vi "CH_LM Calibration Example.vi"() -> ()   [LabVIEW 2012, in "CH_LM.lvlib"]
doc: "This example VI can be used to query or set the calibration paramters."
uses:
  CH_LM.lvlib
  <vilib>/Utility/error.llb/DialogType.ctl
  CH_LM Calibration SlowADC Channel.ctl
  CH_LM ProbeQualifier.ctl
  CH_LM ProbeType.ctl
  CH_LM Meter Type.ctl
  CH_LM System StatusCluster.ctl
  CH_LM Date Format.ctl
panel:
  in  "Update All":bool
  in  "stop":bool
  in  "Unlock? (True)":bool
  out "GUI Loop":i32
  out "Lock timed out":bool
  in  "Reset Error":bool
  out "Event error":errorcluster
  in  "Tab Control":enum32{"Main", "Calibration"}(tab)
  out "Qualifier":T1
  out "Serial Number":string
  out "Head Temperature":dbl[unit]=273.15
  out "Status Description":string
  out "Status":T2
  out "Date Format":T3
  out "Time Stamp":timestamp format="%<%X\n%x>T"
  in  "Update Probe":bool
  out "Responsitivity":dbl format="%#.1g"
  out "Calibration Date":timestamp format="%<%x>T"
  out "Serial Number":string
  out "Probe Type":T4
  out "Probe Model":string
  out "Meter Type":T5
  out "Calibration Date":string
  out "Self-Test Result Message":string
  out "Self-Test Result Code":i32
  out "Date":string
  out "Revision":string
  out "Instrument Driver Revision":string
  out "Vendor":string
  out "Module":string
  out "timed out?":bool
  in  "Address":i32=1
  in  "Serial Number":string
  in  "Reset? (F: No)":bool
  in  "ID Query? (T: Yes)":bool
  in  "PYRO DAC Offset (0)":u16
  out "PYRO DAC Offset":u16
  in  "set Gain & Offset":bool
  in  "read Gain & Offset":bool
  in  "Hardware Calibration":T6={"Pyro DAC Attenuator"=0, "Pyro Input Attenuator"=1, "T Control"=0, "S Control"=0, "G Control"=0, "P Control"=0}
  in  "RTTR":u32=4294967295 format="%.0x"
  in  "Counts at 4V":i32
  in  "Counts at 0V":i32
  in  "DAC counts":i32
  out "Slow ADC value":i32 format="%.0x"
  in  "Slow ADC Channel":T7
  out "ADC value":i32 format="%.0x"
  out "Peak value":i32 format="%.0x"
  in  "set Probe Type":bool
  in  "Responsitivity new":dbl format="%#.1g"
  in  "Probe Type new":T4
  in  "Meter Info":bool
  in  "Calibration Date new":string
  in  "Serial Number new":string
  in  "Meter Type new":T5
  in  "Password":string
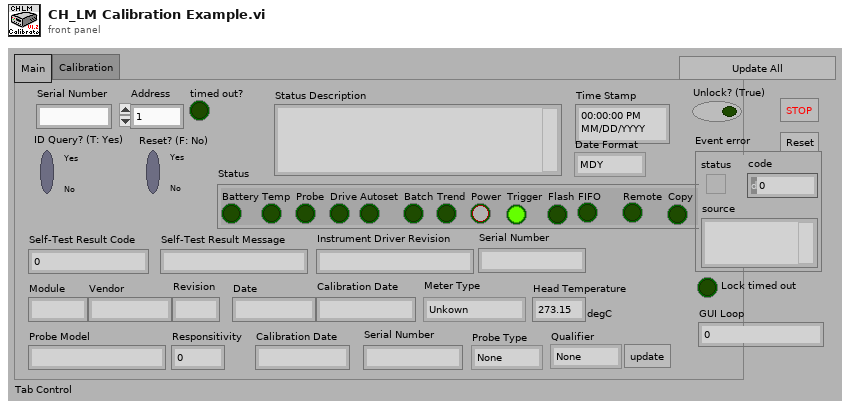
[diagram p1: front panel]
types:
  T1 = typedef "CH_LM.lvlib/CH_LM ProbeQualifier.ctl" = enum16{"None", "Single", "Quad", "No Spec"}
  T2 = typedef "CH_LM.lvlib/CH_LM System StatusCluster.ctl" = cluster{"Battery":bool, "Temp":bool, "Probe":bool, "Drive":bool, "Autoset":bool, "Batch":bool, "Trend":bool, "Power":bool, "Trigger":bool, "Flash":bool, "FIFO":bool, "Remote":bool, "Copy":bool}
  T3 = typedef "CH_LM.lvlib/CH_LM Date Format.ctl" = enum16{"MDY", "DMY"}
  T4 = typedef "CH_LM.lvlib/CH_LM ProbeType.ctl" = enum16{"None", "Thermopile", "Pyroelectric", "Optical"}
  T5 = typedef "CH_LM.lvlib/CH_LM Meter Type.ctl" = enum16{"Unkown", "TOP", "TO"}
  T6 = cluster{"Pyro DAC Attenuator":i32, "Pyro Input Attenuator":i32, "T Control":i32, "S Control":i32, "G Control":i32, "P Control":i32}
  T7 = typedef "CH_LM.lvlib/CH_LM Calibration SlowADC Channel.ctl" = enum16{"Up", "Down", "Left", "Right", "P Max", "L Thermistor", "P Thermistor", "Optical"}
  T8 = typedef "CH_LM.lvlib/CH_LM Calibration Hardware Override.ctl" = cluster{"Pyro DAC Attenuator":i32, "Pyro Input Attenuator":i32, "Q Control":i32, "S Control":i32, "G Control":i32, "P Control":i32}
  T9 = typedef "DialogType.ctl" = u16
  T10 = typedef "CH_LM.lvlib/CH_LM Calibration Data Thermopile.ctl" = cluster{"Range 1.0":T11}
  T11 = typedef "CH_LM.lvlib/CH_LM Calibration Data.ctl" = cluster{"Gain":dbl, "Offset":dbl}
  T12 = typedef "CH_LM.lvlib/CH_LM Calibration Data Pyroelectric.ctl" = cluster{"Range 0.1":T11, "Range 0.2":T11, "Range 0.4":T11, "Range 0.5":T11, "Range 0.8":T11, "Range 1.0":T11, "Range 2.0":T11, "Range 4.0":T11, "Range 5.0":T11, "Range 8.0":T11, "Range 10.0":T11, "Range 20.0":T11, "Range 40.0":T11, "Range 50.0":T11, "Range 80.0":T11, "Range 100.0":T11, "Range 200.0":T11, "Range 400.0":T11, "Range 500.0":T11, "Range 800.0":T11, "Range 1000.0":T11, "Range 2000.0":T11, "Range 4000.0":T11}
  T13 = typedef "CH_LM.lvlib/CH_LM Calibration Data Optical.ctl" = cluster{"Range 68.1 Ohm":T11, "Range 100.0 kOhm":T11}
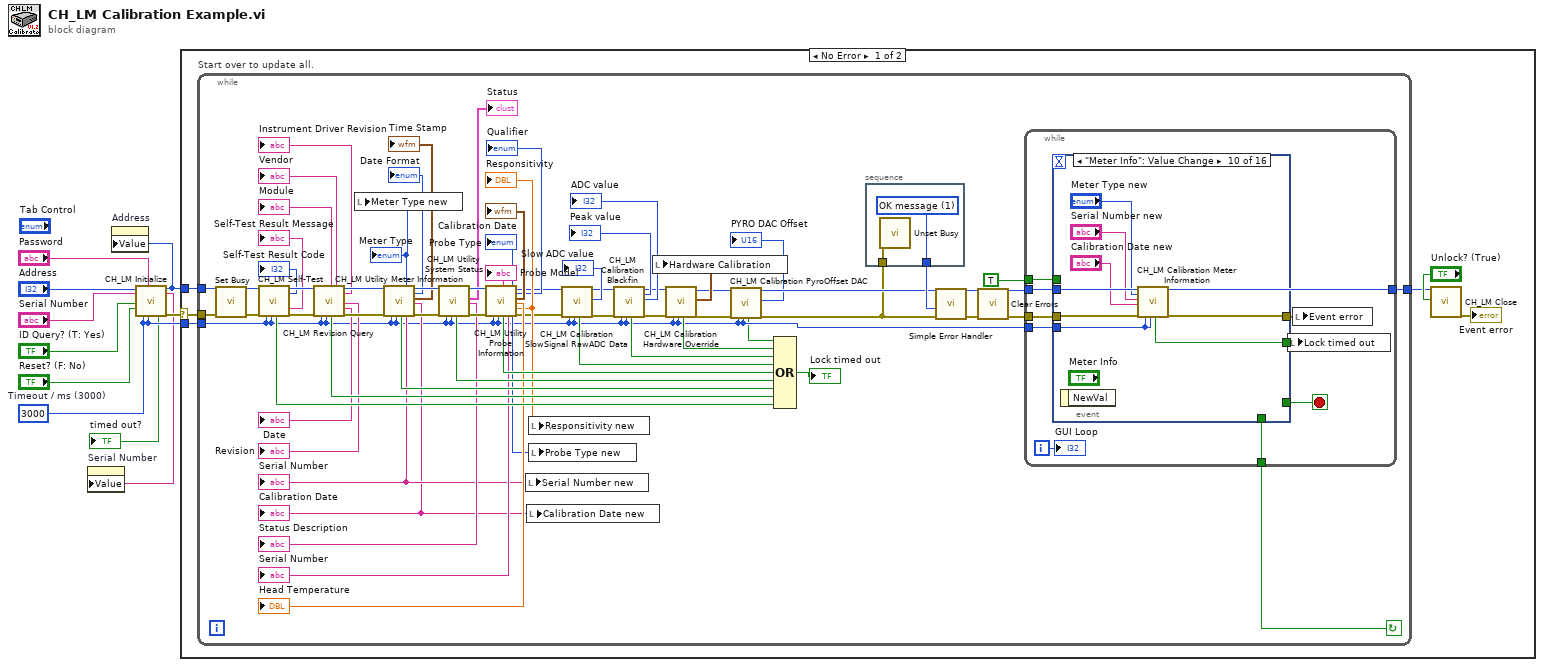
[diagram p0: block diagram]
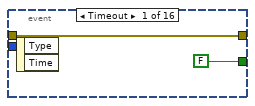
[diagram p2: hidden frame]
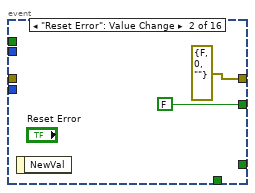
[diagram p3: hidden frame]
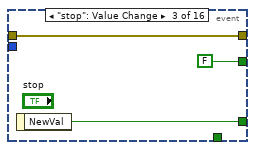
[diagram p4: hidden frame]
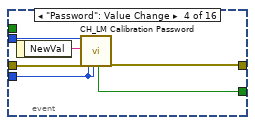
[diagram p5: hidden frame]
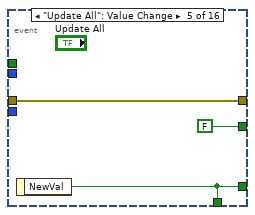
[diagram p6: hidden frame]
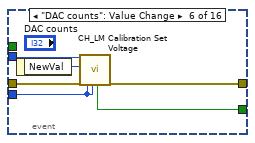
[diagram p7: hidden frame]
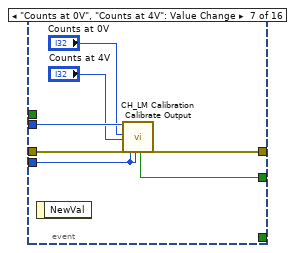
[diagram p8: hidden frame]
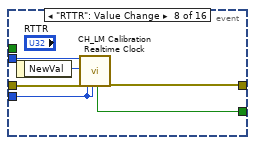
[diagram p9: hidden frame]
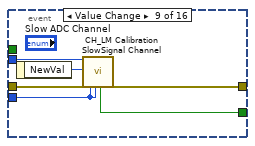
[diagram p10: hidden frame]
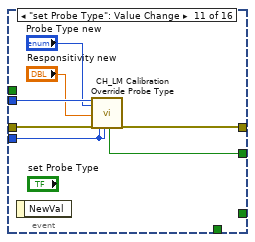
[diagram p11: hidden frame]
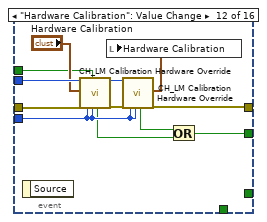
[diagram p12: hidden frame]
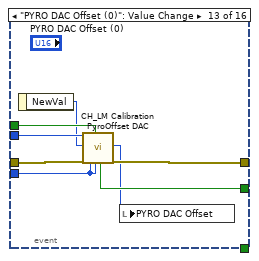
[diagram p13: hidden frame]
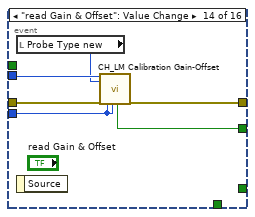
[diagram p14: hidden frame]
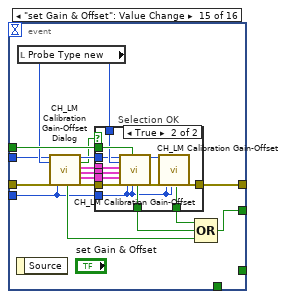
[diagram p15: hidden frame]
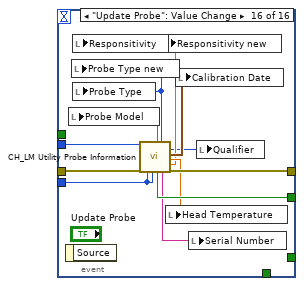
[diagram p17: hidden frame]
diagram:
  w10 = 3000  # Timeout / ms (3000)
  n1 = call "CH_LM Initialize.vi"("Address"="Address", "Serial Number"="Serial Number", "ID Query (True)"="ID Query? (T: Yes)", "Reset (False)"="Reset? (F: No)", "Timeout / ms (3000)"=w10, "Password"="Password", "Lock Timeout / ms (1000)"=w10) -> ("timed out?"=→"timed out?":bool, "Meter Index"=w2:i32, "Serial Number"=w1:string, "error out"=w3:errorcluster)  [unwired: 2 in, 7 out]
  n2 = property on="Serial Number" class="Str"("Value"=w1) -> ()  [unwired: 2 in, 2 out]
  n3 = property on="Address" class="DigNum (strict)"("Value"=w2) -> ()  [unwired: 2 in, 2 out]
  n4 = case shown="No Error" w3 {
    selector: w3 -> [w15 _]
    tunnel: w2 -> [w16 _]
    tunnel: w10 -> [w12 _]
    frame No Error {
      n5 = while "Start over to update all." {
        tunnel: w16 -> [w72]
        tunnel: w15 -> [w41]
        tunnel: w12 -> [w18]
        tunnel: [w49] -> w11
        stop <- w43 continue-if-true
        n6 = call <vilib>:"Set Busy.vi"("error in (no error)"=w41) -> ("error out"=w42:errorcluster)  [unwired: 3 in, 7 out]
        n7 = call "CH_LM Self-Test.vi"("Meter Index"=w72, "error in (no error)"=w42, "Timeout / ms (3000)"=w18, "Lock Timeout / ms (1000)"=w18) -> ("Lock timed out"=w63:bool, "Meter Index"=w73:i32, "Self-Test Result Code"=→"Self-Test Result Code":i32, "Self-Test Result Message"=→"Self-Test Result Message":string, "error out"=w80:errorcluster)  [unwired: 11 out]
        n8 = call "CH_LM Revision Query.vi"("Meter Index"=w73, "error in (no error)"=w80, "Timeout / ms (3000)"=w18, "Lock Timeout / ms (1000)"=w18) -> ("Module"=→"Module":string, "Lock timed out"=w64:bool, "Vendor"=→"Vendor":string, "Meter Index"=w78:i32, "Instrument Driver Revision"=→"Instrument Driver Revision":string, "Instrument Firmware Revision"=→"Revision":string, "Instrument Firmware Date"=→"Date":string, "error out"=w77:errorcluster)  [unwired: 8 out]
        n9 = call "CH_LM Utility Meter Information.vi"("Meter Index"=w78, "error in (no error)"=w77, "Timeout / ms (3000)"=w18, "Lock Timeout / ms (1000)"=w18) -> ("Lock timed out"=w65:bool, "Meter Type"=w48:T5, "Serial Number"=w47:string, "Meter Index"=w79:i32, "Date Format"=→"Date Format":T3, "Time Stamp"=→"Time Stamp":timestamp, "Calibration Date"=w46:string, "error out"=w76:errorcluster)  [unwired: 3 in, 5 out]
        "Meter Type" <- w48
        "Calibration Date" <- w46
        "Serial Number" <- w47
        n10 = local write "Meter Type new"(w48) -> ()
        n11 = call "CH_LM Utility System Status.vi"("Meter Index"=w79, "error in (no error)"=w76, "Timeout / ms (3000)"=w18, "Lock Timeout / ms (1000)"=w18) -> ("Lock timed out"=w66:bool, "Meter Index"=w74:i32, "Status"=→"Status":T2, "Status Description"=→"Status Description":string, "error out"=w75:errorcluster)  [unwired: 11 out]
        n12 = call "CH_LM Utility Probe Information.vi"("Meter Index"=w74, "error in (no error)"=w75, "Timeout / ms (3000)"=w18, "Lock Timeout / ms (1000)"=w18) -> ("Model"=→"Probe Model":string, "Lock timed out"=w67:bool, "Probe Type"=w45:T4, "Serial Number"=→"Serial Number":string, "Meter Index"=w31:i32, "Probe Qualifier"=→"Qualifier":T1, "Calibration Date"=→"Calibration Date":timestamp, "Head Temperature"=→"Head Temperature":dbl[unit], "Responsitivity"=w40:dbl, "error out"=w33:errorcluster)  [unwired: 6 out]
        "Probe Type" <- w45
        "Responsitivity" <- w40
        n13 = local write "Serial Number new"(w47) -> ()
        n14 = local write "Calibration Date new"(w46) -> ()
        n15 = local write "Responsitivity new"(w40) -> ()
        n16 = local write "Probe Type new"(w45) -> ()
        n17 = call "CH_LM Calibration SlowSignal RawADC Data.vi"("Meter Index"=w31, "error in (no error)"=w33, "Timeout / ms (3000)"=w18, "Lock Timeout / ms (1000)"=w18) -> ("Lock timed out"=w32:bool, "Meter Index"=w30:i32, "Slow ADC value"=→"Slow ADC value":i32, "error out"=w29:errorcluster)  [unwired: 12 out]
        n18 = call "CH_LM Calibration Blackfin.vi"("Meter Index"=w30, "error in (no error)"=w29, "Timeout / ms (3000)"=w18, "Lock Timeout / ms (1000)"=w18) -> ("Lock timed out"=w28:bool, "Meter Index"=w27:i32, "Peak value"=→"Peak value":i32, "ADC value"=→"ADC value":i32, "error out"=w26:errorcluster)  [unwired: 11 out]
        n19 = call "CH_LM Calibration Hardware Override.vi"("Meter Index"=w27, "error in (no error)"=w26, "Timeout / ms (3000)"=w18, "Lock Timeout / ms (1000)"=w18) -> ("Lock timed out"=w25:bool, "Meter Index"=w23:i32, "Hardware Calibration"=w37:T8, "error out"=w21:errorcluster)  [unwired: 2 in, 10 out]
        n20 = local write "Hardware Calibration"(w37) -> ()
        n21 = call "CH_LM Calibration PyroOffset DAC.vi"("Meter Index"=w23, "error in (no error)"=w21, "Timeout / ms (3000)"=w18, "Lock Timeout / ms (1000)"=w18) -> ("Lock timed out"=w17:bool, "Meter Index"=w22:i32, "PYRO DAC Offset"=→"PYRO DAC Offset":u16, "error out"=w20:errorcluster)  [unwired: 2 in, 10 out]
        n22 = Compound Arithmetic op=OR(w17, w25, w28, w32, w67, w66, w65, w64, w63) -> (→"Lock timed out":bool)
        n23 = stacked-sequence {
          tunnel: [w82] -> w70
          tunnel: w20 -> [w81]
          frame #0 {
            w82 = T9 1 items=["no dialog", "OK message", "continue or stop message", "OK message + warnings", "continue/stop + warnings"] ("type of dialog (OK msg:1)")
            n24 = call <vilib>:"Unset Busy.vi"("error in (no error)"=w81) -> ()  [unwired: 1 in, 10 out]
          }
        }
        n25 = call <vilib>:"Simple Error Handler.vi"("type of dialog (OK msg:1)"=w70, "error in (no error)"=w20) -> ("error out"=w71:errorcluster)  [unwired: 7 out]
        n26 = call <vilib>:"Clear Errors.vi"("error in (no error)"=w71) -> ("error out"=w50:errorcluster)  [unwired: 1 in, 5 out]
        n27 = while {
          tunnel: w22 -> [w88]
          tunnel: w50 -> [w90]
          tunnel: w18 -> [w85]
          tunnel: [w88] -> w49
          tunnel: TRUE -> [w84]
          tunnel: [w83] -> w43
          i -> [w91]
          stop <- w87 stop-if-true
          n28 = event shown="[9] \"Meter Info\": Value Change" {
            selector: _ -> [_ _ _ _ _ _ _ _ _ _ _ _ _ _ _ _]
            dyn-events: _ -> [_ _ _ _ _ _ _ _ _ _ _ _ _ _ _ _]
            timeout: _ -> [_ _ _ _ _ _ _ _ _ _ _ _ _ _ _ _]
            tunnel: [_ _ w98 _ w105 _ _ _ _ _ _ _ _ _ _ _] -> w87
            tunnel: w88 -> [_ _ _ w104 _ w112 w120 w126 w131 w140 w147 w159 w167 w173 w181 w214]
            tunnel: w90 -> [w93 _ w97 w103 w107 w111 w119 w125 w130 w139 w146 w158 w166 w172 w183 w213]
            tunnel: [w93 errorcluster {"status"=FALSE, "code"=0, "source"=""} ("error out") w97 w101 w107 w108 w116 w123 w127 w134 w144 w153 w165 w171 w189 w207] -> w89
            tunnel: [FALSE FALSE ("Lock timed out") FALSE ("Lock timed out") w100 FALSE ("Lock timed out") w109 w117 w122 w128 w133 w143 w149 w162 w170 w185 w211] -> w86
            tunnel: w85 -> [_ _ _ w99 _ w110 w118 w121 w129 w138 w145 w152 w163 w169 w175 w212]
            tunnel: w84 -> [_ _ _ _ _ _ _ _ _ _ _ w156 w164 _ w188 _]
            tunnel: [_ _ _ _ w105 _ _ _ _ _ _ _ _ _ _ _] -> w83
            event Timeout {
              n29 = event-data() -> ()  [unwired: 3 out]
            }
            event "Reset Error": Value Change {
              n30 = event-data() -> ()  [unwired: 2 out]
            }
            event "stop": Value Change {
              n31 = event-data() -> ("NewVal"=w98:bool)  [unwired: 1 out]
            }
            event "Password": Value Change {
              n32 = event-data() -> ("NewVal"=w102:string)  [unwired: 1 out]
              n33 = call "CH_LM Calibration Password.vi"("Meter Index"=w104, "Password"=w102, "error in (no error)"=w103, "Timeout / ms (3000)"=w99, "Lock Timeout / ms (1000)"=w99) -> ("Lock timed out"=w100:bool, "error out"=w101:errorcluster)  [unwired: 13 out]
            }
            event "Update All": Value Change {
              n34 = event-data() -> ("NewVal"=w105:bool)  [unwired: 1 out]
            }
            event "DAC counts": Value Change {
              n35 = event-data() -> ("NewVal"=w113:i32)  [unwired: 1 out]
              n36 = call "CH_LM Calibration Set Voltage.vi"("Meter Index"=w112, "DAC counts"=w113, "error in (no error)"=w111, "Timeout / ms (3000)"=w110, "Lock Timeout / ms (1000)"=w110) -> ("Lock timed out"=w109:bool, "error out"=w108:errorcluster)  [unwired: 13 out]
            }
            event "Counts at 0V", "Counts at 4V": Value Change {
              n37 = event-data() -> ()  [unwired: 2 out]
              n38 = call "CH_LM Calibration Calibrate Output.vi"("Meter Index"=w120, "Counts at 0V"="Counts at 0V", "Counts at 4V"="Counts at 4V", "error in (no error)"=w119, "Timeout / ms (3000)"=w118, "Lock Timeout / ms (1000)"=w118) -> ("Lock timed out"=w117:bool, "error out"=w116:errorcluster)  [unwired: 12 out]
            }
            event "RTTR": Value Change {
              n39 = event-data() -> ("NewVal"=w124:u32)  [unwired: 1 out]
              n40 = call "CH_LM Calibration Realtime Clock.vi"("Meter Index"=w126, "RTTR"=w124, "error in (no error)"=w125, "Timeout / ms (3000)"=w121, "Lock Timeout / ms (1000)"=w121) -> ("Lock timed out"=w122:bool, "error out"=w123:errorcluster)  [unwired: 13 out]
            }
            event Value Change {
              n41 = event-data() -> ("NewVal"=w132:T7)  [unwired: 1 out]
              n42 = call "CH_LM Calibration SlowSignal Channel.vi"("Meter Index"=w131, "Slow ADC Channel"=w132, "error in (no error)"=w130, "Timeout / ms (3000)"=w129, "Lock Timeout / ms (1000)"=w129) -> ("Lock timed out"=w128:bool, "error out"=w127:errorcluster)  [unwired: 13 out]
            }
            event "Meter Info": Value Change {
              n43 = event-data() -> ()  [unwired: 2 out]
              n44 = call "CH_LM Calibration Meter Information.vi"("Meter Index"=w140, "Meter Type"="Meter Type new", "Serial Number"="Serial Number new", "Calibration Date"="Calibration Date new", "error in (no error)"=w139, "Timeout / ms (3000)"=w138, "Lock Timeout / ms (1000)"=w138) -> ("Lock timed out"=w133:bool, "error out"=w134:errorcluster)  [unwired: 11 out]
            }
            event "set Probe Type": Value Change {
              n45 = event-data() -> ()  [unwired: 2 out]
              n46 = call "CH_LM Calibration Override Probe Type.vi"("Meter Index"=w147, "Probe Type"="Probe Type new", "Responsitivity"="Responsitivity new", "error in (no error)"=w146, "Timeout / ms (3000)"=w145, "Lock Timeout / ms (1000)"=w145) -> ("Lock timed out"=w143:bool, "error out"=w144:errorcluster)  [unwired: 12 out]
            }
            event "Hardware Calibration": Value Change {
              n47 = event-data() -> ()  [unwired: 2 out]
              n48 = call "CH_LM Calibration Hardware Override.vi"("Meter Index"=w159, "Hardware Calibration"="Hardware Calibration", "error in (no error)"=w158, "Timeout / ms (3000)"=w152, "Action (query)"=w156, "Lock Timeout / ms (1000)"=w152) -> ("Lock timed out"=w150:bool, "Meter Index"=w155:i32, "error out"=w154:errorcluster)  [unwired: 11 out]
              n49 = call "CH_LM Calibration Hardware Override.vi"("Meter Index"=w155, "error in (no error)"=w154, "Timeout / ms (3000)"=w152, "Lock Timeout / ms (1000)"=w152) -> ("Lock timed out"=w151:bool, "Hardware Calibration"=w148:T8, "error out"=w153:errorcluster)  [unwired: 2 in, 11 out]
              n50 = local write "Hardware Calibration"(w148) -> ()
              n51 = Or(x=w151, y=w150) -> (x .or. y?=w149:bool)
            }
            event "PYRO DAC Offset (0)": Value Change {
              n52 = event-data() -> ("NewVal"=w161:u16)  [unwired: 1 out]
              n53 = call "CH_LM Calibration PyroOffset DAC.vi"("Meter Index"=w167, "PYRO DAC Offset (0)"=w161, "error in (no error)"=w166, "Timeout / ms (3000)"=w163, "Action (query)"=w164, "Lock Timeout / ms (1000)"=w163) -> ("Lock timed out"=w162:bool, "PYRO DAC Offset"=w160:u16, "error out"=w165:errorcluster)  [unwired: 11 out]
              n54 = local write "PYRO DAC Offset"(w160) -> ()
            }
            event "read Gain & Offset": Value Change {
              n55 = local read "Probe Type new"() -> (w168:T4)
              n56 = event-data() -> ()  [unwired: 2 out]
              n57 = call "CH_LM Calibration Gain-Offset.vi"("Meter Index"=w173, "Probe Type"=w168, "error in (no error)"=w172, "Timeout / ms (3000)"=w169, "Lock Timeout / ms (1000)"=w169) -> ("Lock timed out"=w170:bool, "error out"=w171:errorcluster)  [unwired: 4 in, 9 out]
            }
            event "set Gain & Offset": Value Change {
              n58 = event-data() -> ()  [unwired: 2 out]
              n59 = local read "Probe Type new"() -> (w184:T4)
              n60 = call "CH_LM Calibration Gain-Offset Dialog.vi"("Meter Index"=w181, "Probe Type"=w184, "error in (no error)"=w183, "Timeout / ms (3000)"=w175) -> ("Lock timed out"=w176:bool, "Meter Index"=w180:i32, "OK"=w174:bool, "Thermopile Calibration"=w179:T10, "Pyroelectric Calibration"=w178:T12, "Optical Calibration"=w177:T13, "error out"=w182:errorcluster)  [unwired: 9 out]
              n61 = case "Selection OK" shown="True" w174 {
                tunnel: [w190 w202] -> w189
                tunnel: w188 -> [_ w200]
                tunnel: [_ w199] -> w187
                tunnel: [_ w198] -> w186
                tunnel: w184 -> [_ w197]
                tunnel: w182 -> [w190 w196]
                tunnel: w180 -> [_ w195]
                tunnel: w179 -> [_ w194]
                tunnel: w178 -> [_ w193]
                tunnel: w177 -> [_ w192]
                tunnel: w175 -> [_ w191]
                frame False {
                }
                frame True {
                  n62 = call "CH_LM Calibration Gain-Offset.vi"("Meter Index"=w195, "Probe Type"=w197, "Thermopile Calibration"=w194, "Pyroelectric Calibration"=w193, "Optical Calibration"=w192, "error in (no error)"=w196, "Timeout / ms (3000)"=w191, "Action (query)"=w200, "Lock Timeout / ms (1000)"=w191) -> ("Lock timed out"=w198:bool, "Meter Index"=w201:i32, "error out"=w202:errorcluster)  [unwired: 8 out]
                  n63 = call "CH_LM Calibration Gain-Offset.vi"("Meter Index"=w201, "Timeout / ms (3000)"=w191, "Lock Timeout / ms (1000)"=w191) -> ("Lock timed out"=w199:bool)  [unwired: 6 in, 10 out]
                }
              }
              n64 = Compound Arithmetic op=OR(w187, w186, w176) -> (w185:bool)
            }
            event "Update Probe": Value Change {
              n65 = event-data() -> ()  [unwired: 2 out]
              n66 = call "CH_LM Utility Probe Information.vi"("Meter Index"=w214, "error in (no error)"=w213, "Timeout / ms (3000)"=w212, "Lock Timeout / ms (1000)"=w212) -> ("Model"=w210:string, "Lock timed out"=w211:bool, "Probe Type"=w209:T4, "Serial Number"=w205:string, "Probe Qualifier"=w203:T1, "Calibration Date"=w208:timestamp, "Head Temperature"=w206:dbl[unit], "Responsitivity"=w204:dbl, "error out"=w207:errorcluster)  [unwired: 7 out]
              n67 = local write "Probe Model"(w210) -> ()
              n68 = local write "Probe Type new"(w209) -> ()
              n69 = local write "Responsitivity"(w204) -> ()
              n70 = local write "Probe Type"(w209) -> ()
              n71 = local write "Responsitivity new"(w204) -> ()
              n72 = local write "Head Temperature"(w206) -> ()
              n73 = local write "Calibration Date"(w208) -> ()
              n74 = local write "Serial Number"(w205) -> ()
              n75 = local write "Qualifier"(w203) -> ()
            }
          }
          n76 = local write "Lock timed out"(w86) -> ()
          n77 = local write "Event error"(w89) -> ()
          "GUI Loop" <- w91
        }
      }
      n78 = call "CH_LM Close.vi"("Meter Index"=w11, "Unlock? (True)"="Unlock? (True)") -> ("error out"=→"Event error":errorcluster)  [unwired: 1 in, 16 out]
    }
    frame Error {
    }
  }
